vi "ep_Get Filter Coefficients.vi"(6 "fs [Hz]":dbl=1.0 format="%.2f", 8 "error in (no error)":errorcluster, 9 "filter type":T1, 10 "ripple specs":T2={"passband"=0.1, "stopband"=60.0, "dB/linear? (T: dB)"=TRUE}, 11 "freq specs [Hz]":T3={"fpass 1"=0.2, "fstop 1"=0.3, "fpass 2 "=0.0, "fstop 2"=0.0}) -> (0 "error out":errorcluster, 2 "estimated order":i32, 3 "filter coefficients":dbl[](array[numeric]))   [LabVIEW 2013, in "NI_EP_Resample_Host.lvlib"]
uses:
  <vilib>/addons/Electrical Power/PQ/Resampling/NI_EP_Resample_Host.lvlib
  <vilib>/Analysis/3filter.llb/Filter Passband Type.ctl
  <vilib>/Analysis/4window.llb/windowTd.ctl
  <vilib>/Analysis/NI_AALBase.lvlib
  <vilib>/Analysis/NI_AALPro.lvlib
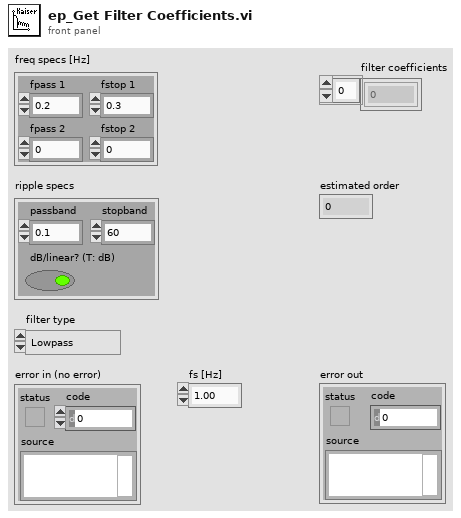
[diagram p1: front panel]
types:
  T1 = typedef "NI_AALBase.lvlib/Filter Passband Type.ctl" = enum32{"Lowpass", "Highpass", "Bandpass", "Bandstop"}
  T2 = cluster{"passband":dbl, "stopband":dbl, "dB/linear? (T: dB)":bool}
  T3 = cluster{"fpass 1":dbl, "fstop 1":dbl, "fpass 2 ":dbl, "fstop 2":dbl}
  T4 = typedef "NI_AALPro.lvlib/windowTd.ctl" = u32
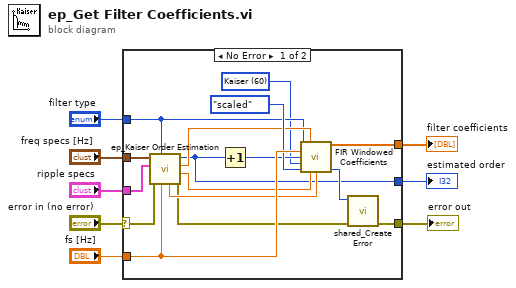
[diagram p0: block diagram]
diagram:
  n1 = case shown="No Error" "error in (no error)" {
    selector: "error in (no error)" -> [w9 w25]
    tunnel: "fs [Hz]" -> [w24 _]
    tunnel: [w22 _] -> w7
    tunnel: "freq specs [Hz]" -> [w21 _]
    tunnel: "ripple specs" -> [w20 _]
    tunnel: [w14 w25] -> w4
    tunnel: "filter type" -> [w13 _]
    tunnel: [w11 _] -> w2
    frame No Error {
      w10 = T4 60 items=["Rectangle"=0, "Hanning"=1, "Hamming"=2, "Blackman-Harris"=3, "Exact Blackman"=4, "Blackman"=5, "Flat Top"=6, "4 Term B-Harris "=7, "7 Term B-Harris"=8, "Low Sidelobe"=9, "Blackman Nuttall"=11, "Triangle"=30, "Bartlett-Hanning"=31, "Bohman"=32, "Parzen"=33, "Welch"=34, "Kaiser"=60, "Dolph-Chebyshev"=61, "Gaussian"=62] ("window")
      n2 = call <vilib>:"ep_Kaiser Order Estimation.vi"("fs [Hz]"=w24, "filter type"=w13, "error in (no error)"=w9, "ripple specs"=w20, "freq specs [Hz]"=w21) -> ("error out"=w15:errorcluster, "low cutoff freq [Hz]"=w18:dbl, "high cutoff freq [Hz]"=w17:dbl, "estimated order"=w11:i32, "beta"=w19:dbl)  [unwired: 2 in]
      n3 = Increment(x=w11) -> (x+1=w12:i32)
      n4 = call <vilib>:"FIR Windowed Coefficients.vi"("filter type"=w13, "high cutoff freq: fh"=w17, "window parameter"=w19, "sampling freq: fs"=w24, "taps"=w12, "window"=w10, "option"=enum32{"not scaled", "scaled"}."scaled", "low cutoff freq: fl"=w18) -> ("FIR Windowed Coefficients"=w22:dbl[], "error"=w16:i32)  [unwired: 6 in]
      n5 = call <vilib>:"shared_Create Error.vi"("error in (no error)"=w15, "error code (0)"=w16) -> ("error out"=w14:errorcluster)  [unwired: 9 in]
    }
    frame Error {
    }
  }
  "filter coefficients" <- w7
  "error out" <- w4
  "estimated order" <- w2
